vi "Teleop.vi"(10 "Match Info":T2={"Autonomous Elapsed Seconds"=0.0, "TeleOp Elapsed Seconds"=0.0, "Disabled Elapsed Seconds"=0.0, "Visited Autonomous"=FALSE, "Visited TeleOp"=FALSE, "Visited Disabled"=FALSE, "Autonomous Settings"={"Autonomous Style"=enum."Independent", "VI Refnum"=refnum}}, 11 "Call Context":T3) -> ()   [LabVIEW 2017]
doc: "This VI is called for each TeleOp packet received from the DS where the robot is not disabled. It is often used to read from the joysticks and update I/O or to update setpoints for timed control loops. It should complete and return within 20 milliseconds or it may miss DS packets."
uses:
  <vilib>/Rock Robotics/WPI/DriverStation/WPI_DriverStationDerivedRobotMode.ctl
  <vilib>/Rock Robotics/WPI/DriverStation/WPI_DriverStationMatch Info.ctl
  <vilib>/Rock Robotics/WPI/ThirdParty/Phoenix-LabVIEW/Motor Controller/Controls/CTRE_Phoenix_MotorControl_ControlMode.ctl
  <vilib>/Rock Robotics/WPI/Utilities/WPI_GetSetVariantRefNum.vi
  <vilib>/Rock Robotics/Network Tables/NT Write Boolean Array.vi
  <vilib>/Rock Robotics/Network Tables/NT Write Numeric Array.vi
  Robot Global Data.vi
  <vilib>/Rock Robotics/WPI/RobotDrive/WPI_RobotDriveMecanumDrive_Cartesian.vi
  <vilib>/Rock Robotics/Network Tables/NT Write Boolean.vi
  <vilib>/Rock Robotics/Network Tables/NT Write Number.vi
panel:
  in  "ARM 1 & 2 INPUTS":T1
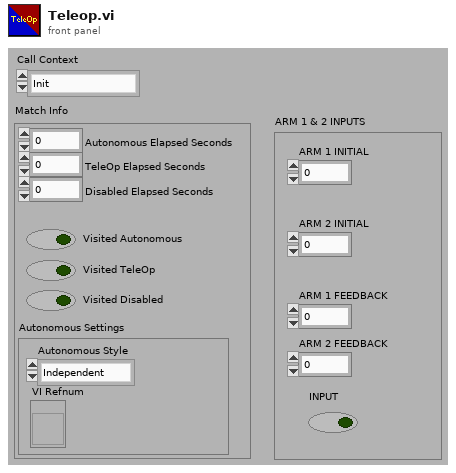
[diagram p1: front panel]
types:
  T1 = cluster{"ARM 1 INITIAL":dbl, "ARM 2 INITIAL":dbl, "ARM 1 FEEDBACK":dbl, "ARM 2 FEEDBACK":dbl, "INPUT":bool}
  T2 = typedef "WPI_DriverStationMatch Info.ctl" = cluster{"Autonomous Elapsed Seconds":dbl, "TeleOp Elapsed Seconds":dbl, "Disabled Elapsed Seconds":dbl, "Visited Autonomous":bool, "Visited TeleOp":bool, "Visited Disabled":bool, "Autonomous Settings":cluster{"Autonomous Style":enum16{"Iterative", "Independent"}, "VI Refnum":refnum<vi>}}
  T3 = typedef "WPI_DriverStationDerivedRobotMode.ctl" = enum16{"Init", "Execute", "Stop"}
  T4 = typedef "CTRE_Phoenix_MotorControl_ControlMode.ctl" = u16
  T5 = typedef "WPI_JoystickDevRef.ctl" = cluster{"Device":T6}
  T6 = typedef "WPI_JoystickDeviceEnum.ctl" = enum16{"USB 0", "USB 1", "USB 2", "USB 3", "USB 4", "USB 5"}
  T7 = cluster{"Axes[0]":dbl, "Axes[1]":dbl, "Axes[2]":dbl, "Axes[3]":dbl, "Axes[4]":dbl, "Axes[5]":dbl, "Axes[6]":dbl, "Axes[7]":dbl, "Axes[8]":dbl}
  T8 = cluster{"Buttons[0]":bool, "Buttons[1]":bool, "Buttons[2]":bool, "Buttons[3]":bool, "Buttons[4]":bool, "Buttons[5]":bool, "Buttons[6]":bool, "Buttons[7]":bool, "Buttons[8]":bool, "Buttons[9]":bool, "Buttons[10]":bool, "Buttons[11]":bool}
  T9 = typedef "WPI_MotorControlDeviceRef.ctl" = cluster{"DeviceStatus":errorcluster, "Type":T10, "PWM":cluster{"PWM Channel":T11, "DeadBand":T12}, "CAN":cluster{"Device Number":u8, "SetOutput VI Ref":variant, "GetOutput VI Ref":variant, "Enable VI Ref":variant, "Disable VI Ref":variant, "Data":variant}, "Invert":bool, "DIO PWM":cluster{"PWM \"Enable\" Channel":T11, "DIOChannel":T13, "PWM Rate":dbl}}
  T10 = typedef "WPI_MotorControlType.ctl" = enum16{"PWM", "CAN", "DIO PWM"}
  T11 = typedef "FPGA_DIOPWMChannel.ctl" = enum8{"PWM 0", "PWM 1", "PWM 2", "PWM 3", "PWM 4", "PWM 5", "PWM 6", "PWM 7", "PWM 8", "PWM 9", "PWM MXP 0", "PWM MXP 1", "PWM MXP 2", "PWM MXP 3", "PWM MXP 4", "PWM MXP 5", "PWM MXP 6", "PWM MXP 7", "PWM MXP 8", "PWM MXP 9", "Invalid"}
  T12 = typedef "WPI_PWMDeadband.ctl" = cluster{"Name":string, "maxPositivePwm":i32, "minPositivePwm":i32, "centerPwm":i32, "maxNegativePwm":i32, "minNegativePwm":i32, "angularRange":u16}
  T13 = typedef "FPGA_DIOChannel.ctl" = enum8{"DIO 0", "DIO 1", "DIO 2", "DIO 3", "DIO 4", "DIO 5", "DIO 6", "DIO 7", "DIO 8", "DIO 9", "DIO MXP 0", "DIO MXP 1", "DIO MXP 2", "DIO MXP 3", "DIO MXP 4", "DIO MXP 5", "DIO MXP 6", "DIO MXP 7", "DIO MXP 8", "DIO MXP 9", "DIO MXP 10", "DIO MXP 11", "DIO MXP 12", "DIO MXP 13", "DIO MXP 14", "DIO MXP 15", "SPI Port CS1", "SPI Port CS2", "SPI Port CS3", "SPI Port MISO", "SPI Port MOSI", "Invalid"}
  T14 = cluster{"Buttons[0]":bool, "Buttons[1]":bool, "Buttons[2]":bool, "Buttons[3]":bool, "Buttons[4]":bool, "Buttons[5]":bool, "Buttons[6]":bool, "Buttons[7]":bool, "Buttons[8]":bool}
  T15 = cluster{"POVs[0]":i16, "POVs[1]":i16, "POVs[2]":i16, "POVs[3]":i16, "POVs[4]":i16, "POVs[5]":i16, "POVs[6]":i16, "POVs[7]":i16, "POVs[8]":i16}
  T16 = typedef "WPI_RobotDriveDevRef.ctl" = cluster{"DevStatus":errorcluster, "Motors[]":T9[], "Square Inputs":bool, "Max Output":dbl}
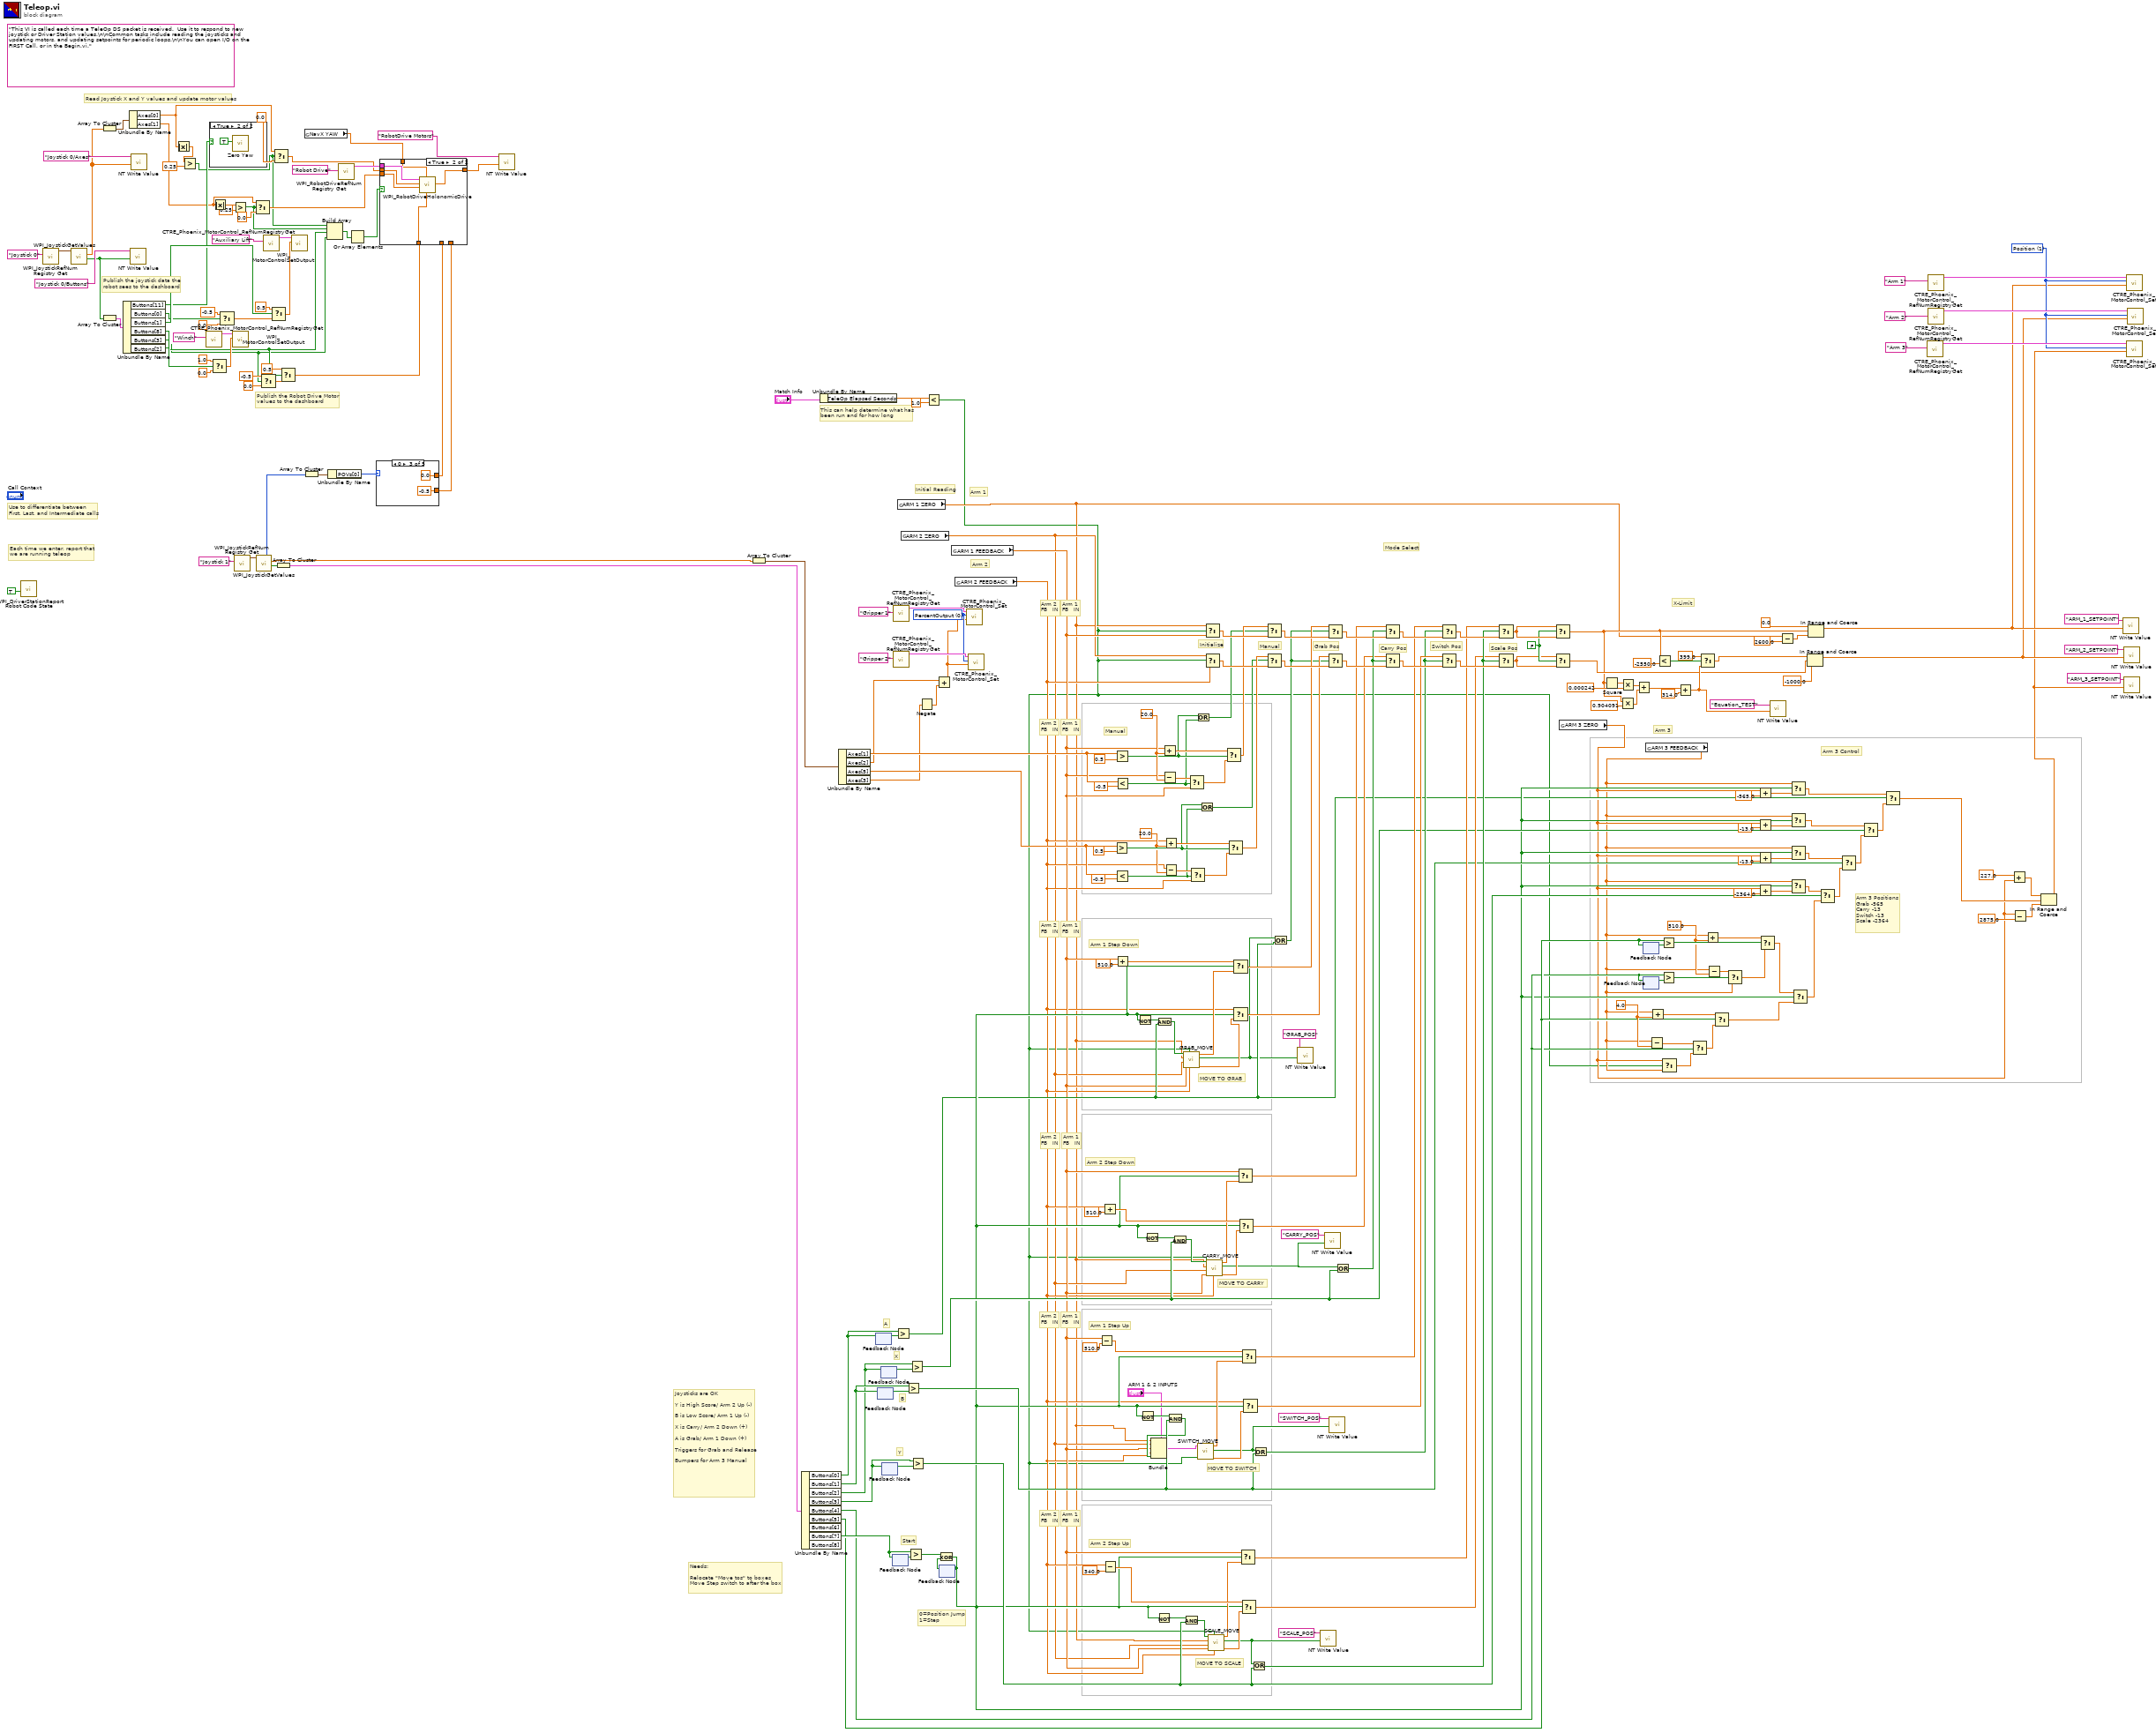
[diagram p0: block diagram]
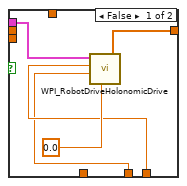
[diagram p2: hidden frame]
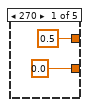
[diagram p3: hidden frame]
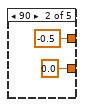
[diagram p4: hidden frame]
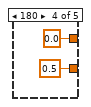
[diagram p5: hidden frame]
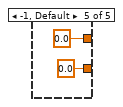
[diagram p6: hidden frame]
diagram:
  w96 = 510.0
  w104 = 4.0
  w109 = FALSE
  w93 = 20.0 ("y")
  w161 = T4 1 items=["PercentOutput"=0, "Position"=1, "Velocity"=2, "Current"=3, "Follower"=5, "MotionProfile"=6, "MotionMagic"=7, "MotionMagicArc"=8, "MotionProfileArc"=10, "Disabled"=15] ("Control Mode")
  w171 = 20.0
  w205 = T4 0 items=["PercentOutput"=0, "Position"=1, "Velocity"=2, "Current"=3, "Follower"=5, "MotionProfile"=6, "MotionMagic"=7, "MotionMagicArc"=8, "MotionProfileArc"=10, "Disabled"=15] ("Control Mode")
  (unwired) "This VI is called each time a TeleOp DS packet is received.  Use it to respond to new joystick or Driver Station values.\n\nCommon tasks include reading the joysticks and updating motors, and updating setpoints for periodic loops.\n\nYou can open I/O on the FIRST Call, or in the Begin.vi."
  # "MOVE TO SCALE"
  # "MOVE TO SWITCH"
  # "MOVE TO CARRY"
  # "MOVE TO GRAB"
  # "Needs:\n\nRelocate \"Move tos\" to boxes\nMove Step switch to after the box"
  # "Arm 3 Positions\nGrab -565\nCarry -13\nSwitch -13\nScale -2364"
  # "Arm 1 Step Down"
  # "Arm 2 Step Down"
  # "Arm 1 Step Up"
  # "Start"
  # "Arm 2 Step Up"
  # "Carry Pos"
  # "Joysticks are OK\n\nY is High Score/ Arm 2 Up (-)\n\nB is Low Score/ Arm 1 Up (-)\n\nX is Carry/ Arm 2 Down (+)\n\nA is Grab/ Arm 1 Down (+)\n\nTriggers for Grab and Release\n\nBumpers for Arm 3 Manual"
  # "Arm 2\nFB   IN"
  # "Arm 1\nFB   IN"
  # "Arm 2\nFB   IN"
  # "Arm 1\nFB   IN"
  # "Arm 2\nFB   IN"
  # "Arm 1\nFB   IN"
  # "Arm 3"
  # "Arm 2"
  # "Arm 1"
  # "Arm 3 Control"
  # "B"
  # "A"
  # "Y"
  # "X"
  # "0=Position Jump\n1=Step"
  # "This can help determine what has\nbeen run and for how long"
  # "Arm 2\nFB   IN"
  # "Arm 1\nFB   IN"
  # "Arm 2\nFB   IN"
  # "Arm 1\nFB   IN"
  # "Manual"
  # "Initial Reading"
  # "Initialize"
  # "Manual"
  # "Grab Pos"
  # "Switch Pos"
  # "Scale Pos"
  # "X-Limit"
  # "Arm 2\nFB   IN"
  # "Arm 1\nFB   IN"
  # "Mode Select"
  # "Publish the Robot Drive Motor\nvalues to the dashboard"
  # "Publish the joystick data the\nrobot sees to the dashboard"
  # "Each time we enter, report that\nwe are running teleop"
  # "Use to differentiate between\nFirst, Last, and Intermediate calls"
  # "Read Joystick X and Y values and update motor values"
  n1 = call <vilib>:"WPI_DriverStationReport Robot Code State.vi"("TeleOp"=TRUE ("Autonomous")) -> ()  [unwired: 10 in, 1 out]
  n2 = call <vilib>:"WPI_JoystickRefNum Registry Get.vi"("refnum name"="Joystick 0") -> ("JoystickDevRef"=w247:T5)  [unwired: 1 in, 9 out]
  n3 = call <vilib>:"WPI_JoystickGetValues.vi"("JoystickDevRef"=w247) -> ("Buttons"=w239:bool[], "Axes"=w241:dbl[])  [unwired: 6 in, 3 out]
  n4 = Array To Cluster(array=w241) -> (cluster=w240:T7)
  n5 = Array To Cluster(array=w239) -> (cluster=w238:T8)
  n6 = Unbundle By Name(w238) -> ("Buttons[11]"=w211:bool, "Buttons[0]"=w234:bool, "Buttons[1]"=w235:bool, "Buttons[8]"=w227:bool, "Buttons[3]"=w23:bool, "Buttons[2]"=w22:bool)
  n7 = Unbundle By Name(w240) -> ("Axes[0]"=w199:dbl, "Axes[1]"=w194:dbl)
  n8 = call-poly <vilib>:"NT Write Value.vi"("Boolean Array"=w239, "Name"="Joystick 0/Buttons") -> ()  [unwired: 9 in, 1 out]
  n9 = call-poly <vilib>:"NT Write Value.vi"("Numeric Array"=w241, "Name"="Joystick 0/Axes") -> ()  [unwired: 9 in, 1 out]
  n10 = Absolute Value(x=w199) -> (abs(x)=w204:dbl)
  n11 = Greater?(x=w204, y=0.25) -> (0:w25:bool)
  n12 = call <vilib>:"CTRE_Phoenix_MotorControl_RefNumRegistryGet.vi"("refnum name"="Winch") -> ("PhoenixMotorControlDevRef"=w221:T9)  [unwired: 9 in, 1 out]
  n13 = case shown="True" w211 {
    frame False {
    }
    frame True {
      n14 = call <vilib>:"Zero Yaw.vi"("Zero"=TRUE) -> ()  [unwired: 11 in]
    }
  }
  n15 = Select(t=1.0, s=w227, f=0.0) -> (s? t:f=w228:dbl)
  n16 = Absolute Value(x=w194) -> (abs(x)=w197:dbl)
  n17 = Select(t=-0.5, s=w234, f=0.0) -> (s? t:f=w233:dbl)
  n18 = call <vilib>:"WPI_MotorControlSetOutput.vi"("Output"=w228, "MotorControlDevRef"=w221) -> ()  [unwired: 7 in, 3 out]
  n19 = Greater?(x=w197, y=0.25) -> (0:w24:bool)
  n20 = call <vilib>:"WPI_JoystickRefNum Registry Get.vi"("refnum name"="Joystick 1") -> ("JoystickDevRef"=w220:T5)  [unwired: 1 in, 9 out]
  n21 = Select(t=w194, s=w24, f=0.0) -> (s? t:f=w198:dbl)
  n22 = call <vilib>:"WPI_JoystickGetValues.vi"("JoystickDevRef"=w220) -> ("Buttons"=w212:bool[], "Axes"=w214:dbl[], "POVs"=w208:i16[])  [unwired: 6 in, 2 out]
  n23 = Select(t=-0.5, s=w22, f=0.0) -> (s? t:f=w144:dbl)
  n24 = call <vilib>:"CTRE_Phoenix_MotorControl_RefNumRegistryGet.vi"("refnum name"="Auxiliary Lift") -> ("PhoenixMotorControlDevRef"=w236:T9)  [unwired: 9 in, 1 out]
  n25 = Select(t=0.5, s=w235, f=w233) -> (s? t:f=w229:dbl)
  n26 = Select(t=w199, s=w25, f=0.0) -> (s? t:f=w201:dbl)
  n27 = Array To Cluster(array=w212) -> (cluster=w213:T14)
  n28 = Select(t=0.5, s=w23, f=w144) -> (s? t:f=w145:dbl)
  n29 = call <vilib>:"WPI_MotorControlSetOutput.vi"("Output"=w229, "MotorControlDevRef"=w236) -> ()  [unwired: 7 in, 3 out]
  n30 = Array To Cluster(array=w208) -> (cluster=w209:T15)
  n31 = global read "Robot Global Data.vi" "NavX YAW"() -> (w12:dbl)
  n32 = Build Array(w25, w24, w23, w22) -> (w21:bool[])
  n33 = Unbundle By Name(w209) -> ("POVs[0]"=w210:i16)
  n34 = call <vilib>:"WPI_RobotDriveRefNum Registry Get.vi"("refnum name"="Robot Drive") -> ("RobotDriveDevRef"=w249:T16)  [unwired: 1 in, 9 out]
  n35 = Or Array Elements(Boolean array=w21) -> (logical OR=w26:bool)
  n36 = case shown="0" w210 {
    tunnel: [0.5 -0.5 0.0 0.0 0.0] -> w16
    tunnel: [0.0 0.0 -0.5 0.5 0.0] -> w15
    frame 270 {
    }
    frame 90 {
    }
    frame 0 {
    }
    frame 180 {
    }
    frame -1, Default {
    }
  }
  n37 = case shown="True" w26 {
    tunnel: w249 -> [w265 w271]
    tunnel: [w264 w270] -> w243
    tunnel: w201 -> [_ w269]
    tunnel: w198 -> [_ w268]
    tunnel: w145 -> [_ w267]
    tunnel: w16 -> [w261 _]
    tunnel: w15 -> [w262 _]
    tunnel: w12 -> [_ w266]
    frame False {
      n38 = call-poly <vilib>:"WPI_RobotDriveHolonomicDrive.vi"("Rotation"=0.0, "Y"=w261, "X"=w262, "RobotDriveDevRef"=w265) -> ("Motor Values"=w264:dbl[])  [unwired: 5 in, 2 out]
    }
    frame True {
      n39 = call-poly <vilib>:"WPI_RobotDriveHolonomicDrive.vi"("Rotation"=w267, "Gyro Angle"=w266, "Y"=w268, "X"=w269, "RobotDriveDevRef"=w271) -> ("Motor Values"=w270:dbl[])  [unwired: 4 in, 2 out]
    }
  }
  n40 = call-poly <vilib>:"NT Write Value.vi"("Numeric Array"=w243, "Name"="RobotDrive Motors") -> ()  [unwired: 9 in, 1 out]
  n41 = Array To Cluster(array=w214) -> (cluster=w215:T7)
  n42 = Unbundle By Name(w213) -> ("Buttons[0]"=w121:bool, "Buttons[1]"=w120:bool, "Buttons[2]"=w119:bool, "Buttons[3]"=w118:bool, "Buttons[4]"=w88:bool, "Buttons[5]"=w95:bool, "Buttons[7]"=w153:bool)  [unwired: 2 out]
  n43 = Unbundle By Name("Match Info") -> ("TeleOp Elapsed Seconds"=w3:dbl)
  n44 = Unbundle By Name(w215) -> ("Axes[1]"=w108:dbl, "Axes[2]"=w18:dbl, "Axes[5]"=w166:dbl, "Axes[3]"=w17:dbl)
  n45 = feedback #1() -> (w158:bool)  [unwired: 1 in]
  n46 = feedback-in #1(w121) -> ()
  n47 = feedback #2() -> (w157:bool)  [unwired: 1 in]
  n48 = feedback-in #2(w120) -> ()
  n49 = feedback-in #3(w119) -> ()
  n50 = feedback #3() -> (w160:bool)  [unwired: 1 in]
  n51 = feedback #4() -> (w159:bool)  [unwired: 1 in]
  n52 = feedback-in #4(w118) -> ()
  n53 = feedback #5() -> (w156:bool)  [unwired: 1 in]
  n54 = feedback-in #5(w153) -> ()
  n55 = call <vilib>:"CTRE_Phoenix_MotorControl_RefNumRegistryGet.vi"("refnum name"="Gripper 1") -> ("PhoenixMotorControlDevRef"=w207:T9)  [unwired: 9 in, 1 out]
  n56 = call <vilib>:"CTRE_Phoenix_MotorControl_RefNumRegistryGet.vi"("refnum name"="Gripper 2") -> ("PhoenixMotorControlDevRef"=w206:T9)  [unwired: 9 in, 1 out]
  n57 = Greater?(x=w121, y=w158) -> (0:w28:bool)
  n58 = global read "Robot Global Data.vi" "ARM 1 ZERO"() -> (w4:dbl)
  n59 = global read "Robot Global Data.vi" "ARM 2 ZERO"() -> (w5:dbl)
  n60 = Greater?(x=w120, y=w157) -> (0:w36:bool)
  n61 = Greater?(x=w153, y=w156) -> (0:w155:bool)
  n62 = Greater?(x=w119, y=w160) -> (0:w34:bool)
  n63 = Greater?(x=w118, y=w159) -> (0:w39:bool)
  n64 = Negate(x=w17) -> (-x=w20:dbl)
  n65 = Less?(x=w3, y=1.0) -> (x < y?=w1:bool)
  n66 = Add(x=w18, y=w20) -> (x+y=w19:dbl)
  n67 = feedback #6() -> (w154:bool)  [unwired: 1 in]
  n68 = Exclusive Or(1:w154, 2:w155) -> (0:w31:bool)
  n69 = feedback-in #6(w31) -> ()
  n70 = global read "Robot Global Data.vi" "ARM 1 FEEDBACK"() -> (w8:dbl)
  n71 = global read "Robot Global Data.vi" "ARM 2 FEEDBACK"() -> (w7:dbl)
  n72 = call <vilib>:"CTRE_Phoenix_MotorControl_Set.vi"("Output"=w19, "Control Mode"=w205, "PhoenixMotorControlDevRef"=w207) -> ()  [unwired: 7 in, 2 out]
  n73 = call <vilib>:"CTRE_Phoenix_MotorControl_Set.vi"("Output"=w19, "Control Mode"=w205, "PhoenixMotorControlDevRef"=w206) -> ()  [unwired: 7 in, 2 out]
  n74 = Subtract(x=w8, y=510.0) -> (x-y=w112:dbl)
  n75 = Add(x=w7, y=510.0) -> (x+y=w113:dbl)
  n76 = Subtract(x=w7, y=340.0) -> (x-y=w111:dbl)
  n77 = Greater?(x=w166, y=0.5) -> (0:w139:bool)
  n78 = Greater?(x=w108, y=0.5) -> (0:w138:bool)
  n79 = Less?(x=w166, y=-0.5) -> (x < y?=w89:bool)
  n80 = Less?(x=w108, y=-0.5) -> (x < y?=w137:bool)
  n81 = Add(x=w8, y=510.0) -> (x+y=w116:dbl)
  n82 = Not(x=w31) -> (.not. x?=w32:bool)
  n83 = Not(x=w31) -> (.not. x?=w37:bool)
  n84 = Not(x=w31) -> (.not. x?=w35:bool)
  n85 = Not(x=w31) -> (.not. x?=w40:bool)
  n86 = And(x=w32, y=w28) -> (x .and. y?=w30:bool)
  n87 = Add(x=w8, y=w171) -> (x+y=w183:dbl)
  n88 = Subtract(x=w8, y=w171) -> (x-y=w182:dbl)
  n89 = Add(x=w7, y=w93) -> (x+y=w180:dbl)
  n90 = Subtract(x=w7, y=w93) -> (x-y=w179:dbl)
  n91 = And(x=w37, y=w36) -> (x .and. y?=w9:bool)
  n92 = Bundle(cluster="ARM 1 & 2 INPUTS", "ARM 1 INITIAL"=w4, "ARM 2 INITIAL"=w5, "ARM 1 FEEDBACK"=w8, "ARM 2 FEEDBACK"=w7, "INPUT"=w9) -> (w10:T1)
  n93 = And(x=w35, y=w34) -> (x .and. y?=w33:bool)
  n94 = call "GRAB_MOVE.vi"("ARM 2 FEEDBACK"=w7, "RESET"=w1, "ARM 1 FEEDBACK"=w8, "ARM 2 INITIAL IN"=w5, "ARM 1 INITIAL"=w4, "INPUT"=w30) -> ("ARM 2 SETPOINT OUT"=w29:dbl, "RUNNING?"=w27:bool, "ARM 1 SETPOINT OUT"=w67:dbl)  [unwired: 3 in]
  n95 = And(x=w40, y=w39) -> (x .and. y?=w38:bool)
  n96 = Select(t=w182, s=w137, f=w8) -> (s? t:f=w181:dbl)
  n97 = Select(t=w179, s=w89, f=w7) -> (s? t:f=w178:dbl)
  n98 = Or(x=w138, y=w137) -> (x .or. y?=w175:bool)
  n99 = call "SWITCH_MOVE.vi"("RESET"=w1, "ARM 1 & 2 INPUTS"=w10) -> ("ARM 2 SETPOINT OUT"=w54:dbl, "RUNNING?"=w49:bool, "ARM 1 SETPOINT OUT"=w55:dbl)  [unwired: 7 in]
  n100 = Or(x=w139, y=w89) -> (x .or. y?=w174:bool)
  n101 = Select(t=w4, s=w1, f=w8) -> (s? t:f=w185:dbl)
  n102 = Select(t=w5, s=w1, f=w7) -> (s? t:f=w184:dbl)
  n103 = call "CARRY_MOVE.vi"("ARM 2 FEEDBACK"=w7, "RESET"=w1, "ARM 1 FEEDBACK"=w8, "ARM 2 INITIAL"=w5, "ARM 1 INITIAL"=w4, "INPUT"=w33) -> ("ARM 2 SETPOINT OUT"=w62:dbl, "RUNNING?"=w56:bool, "ARM 1 SETPOINT OUT"=w63:dbl)  [unwired: 3 in]
  n104 = call "SCALE_MOVE.vi"("ARM 2 FEEDBACK"=w7, "RESET"=w1, "ARM 1 FEEDBACK"=w8, "ARM 2 INITIAL"=w5, "ARM 1 INITIAL"=w4, "INPUT"=w38) -> ("ARM 2 SETPOINT OUT"=w46:dbl, "RUNNING?"=w45:bool, "ARM 1 SETPOINT OUT"=w47:dbl)  [unwired: 3 in]
  n105 = Select(t=w183, s=w138, f=w181) -> (s? t:f=w177:dbl)
  n106 = Select(t=w180, s=w139, f=w178) -> (s? t:f=w176:dbl)
  n107 = Select(t=w116, s=w31, f=w67) -> (s? t:f=w66:dbl)
  n108 = Select(t=w7, s=w31, f=w29) -> (s? t:f=w65:dbl)
  n109 = Select(t=w8, s=w31, f=w63) -> (s? t:f=w58:dbl)
  n110 = Select(t=w113, s=w31, f=w62) -> (s? t:f=w57:dbl)
  n111 = Select(t=w8, s=w31, f=w47) -> (s? t:f=w43:dbl)
  n112 = Select(t=w111, s=w31, f=w46) -> (s? t:f=w42:dbl)
  n113 = Select(t=w112, s=w31, f=w55) -> (s? t:f=w53:dbl)
  n114 = Select(t=w7, s=w31, f=w54) -> (s? t:f=w52:dbl)
  n115 = Or(x=w45, y=w39) -> (x .or. y?=w44:bool)
  n116 = Or(x=w49, y=w36) -> (x .or. y?=w51:bool)
  n117 = Select(t=w177, s=w175, f=w185) -> (s? t:f=w117:dbl)
  n118 = Select(t=w176, s=w174, f=w184) -> (s? t:f=w76:dbl)
  n119 = Or(x=w27, y=w28) -> (x .or. y?=w64:bool)
  n120 = call-poly <vilib>:"NT Write Value.vi"("Boolean"=w27, "Name"="GRAB_POS") -> ()  [unwired: 9 in, 1 out]
  n121 = call-poly <vilib>:"NT Write Value.vi"("Boolean"=w45, "Name"="SCALE_POS") -> ()  [unwired: 9 in, 1 out]
  n122 = call-poly <vilib>:"NT Write Value.vi"("Boolean"=w56, "Name"="CARRY_POS") -> ()  [unwired: 9 in, 1 out]
  n123 = Select(t=w66, s=w64, f=w117) -> (s? t:f=w190:dbl)
  n124 = Select(t=w65, s=w64, f=w76) -> (s? t:f=w77:dbl)
  n125 = call-poly <vilib>:"NT Write Value.vi"("Boolean"=w49, "Name"="SWITCH_POS") -> ()  [unwired: 9 in, 1 out]
  n126 = Or(x=w56, y=w34) -> (x .or. y?=w59:bool)
  n127 = Select(t=w58, s=w59, f=w190) -> (s? t:f=w189:dbl)
  n128 = Select(t=w57, s=w59, f=w77) -> (s? t:f=w187:dbl)
  n129 = Select(t=w53, s=w51, f=w189) -> (s? t:f=w188:dbl)
  n130 = Select(t=w52, s=w51, f=w187) -> (s? t:f=w186:dbl)
  n131 = Select(t=w43, s=w44, f=w188) -> (s? t:f=w110:dbl)
  n132 = Select(t=w42, s=w44, f=w186) -> (s? t:f=w13:dbl)
  n133 = Select(t=w110, s=w109, f=w110) -> (s? t:f=w41:dbl)
  n134 = Select(t=w13, s=w109, f=w13) -> (s? t:f=w78:dbl)
  n135 = global read "Robot Global Data.vi" "ARM 3 ZERO"() -> (w14:dbl)
  n136 = Square(x=w41) -> (x^2=w136:dbl)
  n137 = Multiply(x=w41, y=0.904091) -> (x*y=w133:dbl)
  n138 = Multiply(x=w136, y=0.000242) -> (x*y=w134:dbl)
  n139 = Add(x=w134, y=w133) -> (x+y=w131:dbl)
  n140 = feedback #7() -> (w103:bool)  [unwired: 1 in]
  n141 = feedback-in #7(w95) -> ()
  n142 = feedback #8() -> (w102:bool)  [unwired: 1 in]
  n143 = feedback-in #8(w88) -> ()
  n144 = global read "Robot Global Data.vi" "ARM 3 FEEDBACK"() -> (w11:dbl)
  n145 = Subtract(x=w11, y=w104) -> (x-y=w106:dbl)
  n146 = Add(x=w11, y=w104) -> (x+y=w105:dbl)
  n147 = Less?(x=w41, y=-2550.0) -> (x < y?=w124:bool)
  n148 = Greater?(x=w95, y=w103) -> (0:w99:bool)
  n149 = Greater?(x=w88, y=w102) -> (0:w98:bool)
  n150 = Select(t=w14, s=w1, f=w11) -> (s? t:f=w91:dbl)
  n151 = Add(x=w131, y=314.0) -> (x+y=w127:dbl)
  n152 = Select(t=w106, s=w88, f=w91) -> (s? t:f=w107:dbl)
  n153 = Select(t=399.0, s=w124, f=w127) -> (s? t:f=w126:dbl)
  n154 = Add(x=w11, y=w96) -> (x+y=w100:dbl)
  n155 = Subtract(x=w11, y=w96) -> (x-y=w97:dbl)
  n156 = Select(t=w105, s=w95, f=w107) -> (s? t:f=w90:dbl)
  n157 = Select(t=w97, s=w98, f=w11) -> (s? t:f=w101:dbl)
  n158 = Add(x=w14, y=-565.0) -> (x+y=w70:dbl)
  n159 = Add(x=w14, y=-13.0) -> (x+y=w71:dbl)
  n160 = Add(x=w14, y=-13.0) -> (x+y=w73:dbl)
  n161 = Add(x=w14, y=-2364.0) -> (x+y=w75:dbl)
  n162 = Select(t=w100, s=w99, f=w101) -> (s? t:f=w94:dbl)
  n163 = call-poly <vilib>:"NT Write Value.vi"("Numeric"=w127, "Name"="Equation_TEST") -> ()  [unwired: 9 in, 1 out]
  n164 = Subtract(x=w4, y=2600.0) -> (x-y=w150:dbl)
  n165 = Select(t=w11, s=w31, f=w70) -> (s? t:f=w69:dbl)
  n166 = Select(t=w11, s=w31, f=w71) -> (s? t:f=w68:dbl)
  n167 = Select(t=w11, s=w31, f=w73) -> (s? t:f=w72:dbl)
  n168 = Select(t=w11, s=w31, f=w75) -> (s? t:f=w74:dbl)
  n169 = Select(t=w94, s=w31, f=w90) -> (s? t:f=w83:dbl)
  n170 = In Range and Coerce(upper limit=w126, x=w78, lower limit=-1000.0) -> (coerced(x)=w122:dbl)  [unwired: 1 out]
  n171 = In Range and Coerce(upper limit=0.0, x=w41, lower limit=w150) -> (coerced(x)=w140:dbl)  [unwired: 1 out]
  n172 = Select(t=w74, s=w39, f=w83) -> (s? t:f=w87:dbl)
  n173 = Select(t=w72, s=w36, f=w87) -> (s? t:f=w86:dbl)
  n174 = Select(t=w68, s=w34, f=w86) -> (s? t:f=w85:dbl)
  n175 = Select(t=w69, s=w28, f=w85) -> (s? t:f=w84:dbl)
  n176 = call <vilib>:"CTRE_Phoenix_MotorControl_RefNumRegistryGet.vi"("refnum name"="Arm 3") -> ("PhoenixMotorControlDevRef"=w191:T9)  [unwired: 9 in, 1 out]
  n177 = call <vilib>:"CTRE_Phoenix_MotorControl_RefNumRegistryGet.vi"("refnum name"="Arm 1") -> ("PhoenixMotorControlDevRef"=w193:T9)  [unwired: 9 in, 1 out]
  n178 = call <vilib>:"CTRE_Phoenix_MotorControl_RefNumRegistryGet.vi"("refnum name"="Arm 2") -> ("PhoenixMotorControlDevRef"=w192:T9)  [unwired: 9 in, 1 out]
  n179 = Add(x=227.0, y=w14) -> (x+y=w148:dbl)
  n180 = Subtract(x=w14, y=2875.0) -> (x-y=w146:dbl)
  n181 = In Range and Coerce(upper limit=w148, x=w84, lower limit=w146) -> (coerced(x)=w92:dbl)  [unwired: 1 out]
  n182 = call-poly <vilib>:"NT Write Value.vi"("Numeric"=w140, "Name"="ARM_1_SETPOINT") -> ()  [unwired: 9 in, 1 out]
  n183 = call-poly <vilib>:"NT Write Value.vi"("Numeric"=w122, "Name"="ARM_2_SETPOINT") -> ()  [unwired: 9 in, 1 out]
  n184 = call-poly <vilib>:"NT Write Value.vi"("Numeric"=w92, "Name"="ARM_3_SETPOINT") -> ()  [unwired: 9 in, 1 out]
  n185 = call <vilib>:"CTRE_Phoenix_MotorControl_Set.vi"("Output"=w140, "Control Mode"=w161, "PhoenixMotorControlDevRef"=w193) -> ()  [unwired: 7 in, 2 out]
  n186 = call <vilib>:"CTRE_Phoenix_MotorControl_Set.vi"("Output"=w92, "Control Mode"=w161, "PhoenixMotorControlDevRef"=w191) -> ()  [unwired: 7 in, 2 out]
  n187 = call <vilib>:"CTRE_Phoenix_MotorControl_Set.vi"("Output"=w122, "Control Mode"=w161, "PhoenixMotorControlDevRef"=w192) -> ()  [unwired: 7 in, 2 out]
